vi "Autonomous Independent.vi"   [LabVIEW 2014]
doc: "This VI is called when autonomous begins, and will automatically be terminated when autonomous ends. You can carry out timed or sensor driven robot movement independently without needing to return to the caller."
uses:
  <vilib>/Rock Robotics/WPI/SafetyOutput/WPI_SafetyOutputConfigMenu.ctl
  <vilib>/Rock Robotics/Network Tables/SD Read Number.vi
  Robot Global Data.vi
  <vilib>/Rock Robotics/WPI/RobotDrive/WPI_RobotDriveGetSetRefNum.vi
types:
  T1 = enum16{"Wait 0", "Reta 1", "Wait 1", "Curva 1 ", "Reta 2", "Curva 2", "Reta 3"}
  T2 = enum16{"Get Bin", "Get Tote", "Wait 1", "Release"}
  T3 = typedef "WPI_SafetyOutputConfigMenu.ctl" = enum16{"Enable", "Disable"}
  T4 = enum16{"FALCOOOOOOOON PUNCH 1", "Wait 1", "FALCOOOOOOOON PUNCH 2", "Wait 2"}
  T5 = enum16{"Wait 0", "Reta 1", "Wait 1", "Reta 2", "Wait 2", "Curva 1", "Wait 3", "Reta 3", "Curva 2", "Wait 4", "Reta 4"}
  T6 = enum16{"Get 1st Tote", "Wait 1", "Get 2nd Tote", "Wait 2", "Get 3rd Tote", "Wait 3", "Release"}
  T7 = enum16{"Wait", "Empty state", "Get Bin", "Get Tote First", "Get Knocked Bin", "Close Gripper - Bin", "Close Gripper", "Carry Bin Mode", "Carry Tote Mode", "Get Tote", "Change Height", "Open Gripper", "Get to 0", "Release Pile"}
  T8 = typedef "WPI_EncoderDevRef.ctl" = cluster{"DevStatus":errorcluster, "EncoderIndex":T9, "CounterIndex":T10, "DistancePerCount":dbl, "Decoding Type":T11}
  T9 = typedef "FPGA_EncoderIdx.ctl" = enum8{"Enc 0", "Enc 1", "Enc 2", "Enc 3", "Enc 4", "Enc 5", "Enc 6", "Enc 7", "Invalid"}
  T10 = typedef "FPGA_CounterCtrSystemIndex.ctl" = enum8{"Ctr 0", "Ctr 1", "Ctr 2", "Ctr 3", "Ctr 4", "Ctr 5", "Ctr 6", "Ctr 7", "Invalid"}
  T11 = typedef "WPI_EncoderType.ctl" = enum16{"1x", "2x", "4x"}
  T12 = typedef "WPI_RobotDriveDevRef.ctl" = cluster{"DevStatus":errorcluster, "Motors[]":T13[], "Square Inputs":bool, "Max Output":dbl}
  T13 = typedef "WPI_MotorControlDeviceRef.ctl" = cluster{"DeviceStatus":errorcluster, "Type":T14, "PWM":cluster{"Controller":T15, "PWM Channel":T16, "DeadBand":T17}, "CAN":cluster{"Device Number":u8, "Control Mode":T18, "Semaphore":T19, "Max Vout":dbl, "TalonSRX Control Mode":T20}, "Invert":bool, "TransformRef":T21, "InvTransformRef":T21}
  T14 = typedef "WPI_MotorControlType.ctl" = enum16{"PWM", "CAN", "CANTalonSRX"}
  T15 = typedef "FPGA_TypedefDigitalModule.ctl" = enum16{"Controller 1"}
  T16 = typedef "FPGA_DIOPWMChannel.ctl" = enum8{"PWM 0", "PWM 1", "PWM 2", "PWM 3", "PWM 4", "PWM 5", "PWM 6", "PWM 7", "PWM 8", "PWM 9", "PWM MXP 0", "PWM MXP 1", "PWM MXP 2", "PWM MXP 3", "PWM MXP 4", "PWM MXP 5", "PWM MXP 6", "PWM MXP 7", "PWM MXP 8", "PWM MXP 9", "Invalid"}
  T17 = typedef "WPI_PWMDeadband.ctl" = cluster{"Name":string, "maxPositivePwm":i32, "minPositivePwm":i32, "centerPwm":i32, "maxNegativePwm":i32, "minNegativePwm":i32, "angularRange":u16}
  T18 = typedef "WPI_CANJaguar_ControlMode.ctl" = enum8{"Percent VBus", "Current", "Speed", "Position", "Voltage"}
  T19 = typedef "Semaphore RefNum" = refnum<k1>
  T20 = typedef "WPI_CANTalonSRX_APIControlMode.ctl" = enum8{"Percent VBus", "Speed", "Position", "Slave", "Unchanged / Invalid"}
  T21 = typedef "WPI_PWMTransform_ConPane.ctl" = refnum<vi>
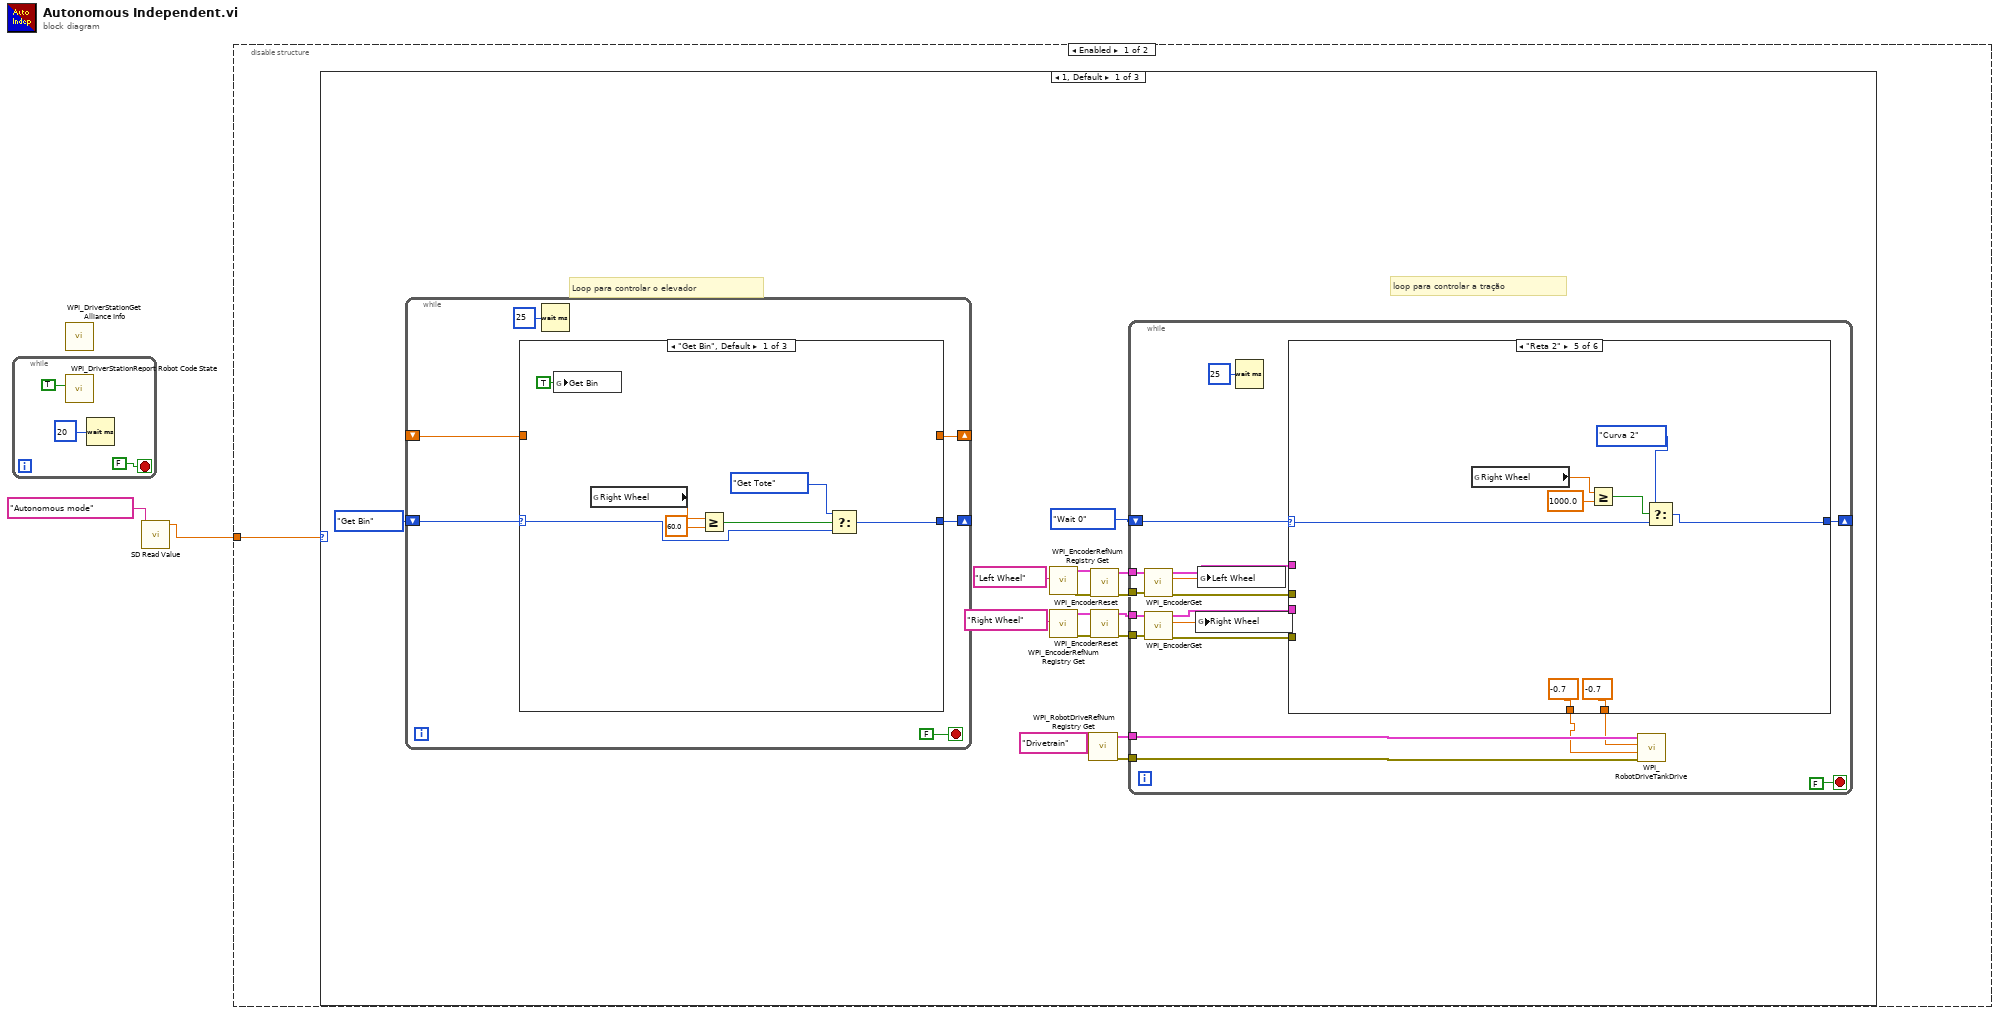
[diagram p0: block diagram]
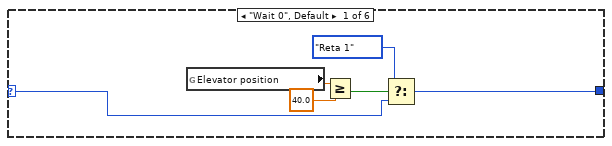
[diagram p2: hidden frame]
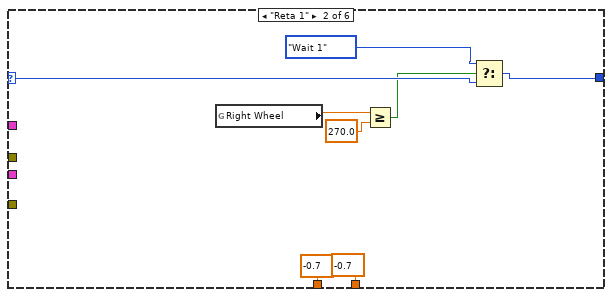
[diagram p3: hidden frame]
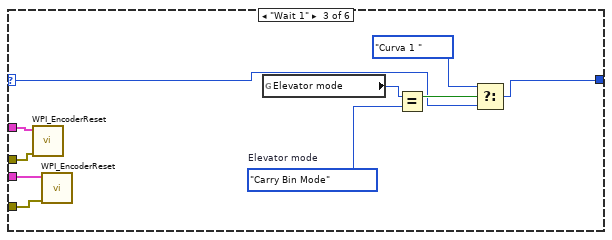
[diagram p4: hidden frame]
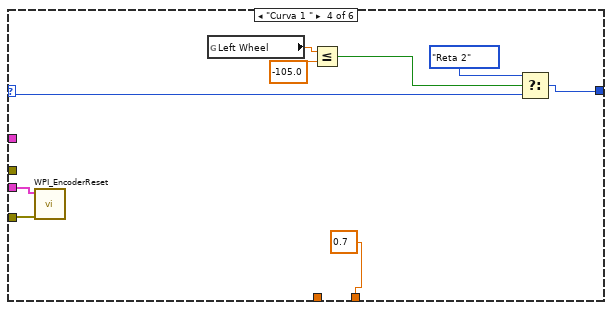
[diagram p5: hidden frame]
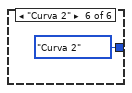
[diagram p6: hidden frame]
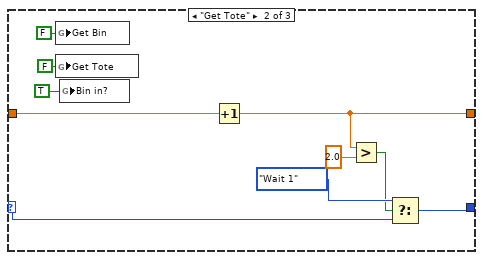
[diagram p7: hidden frame]
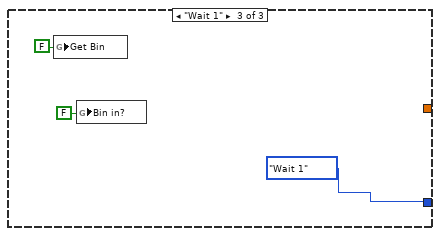
[diagram p8: hidden frame]
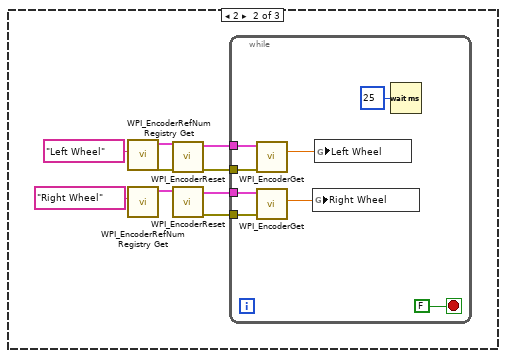
[diagram p9: hidden frame]
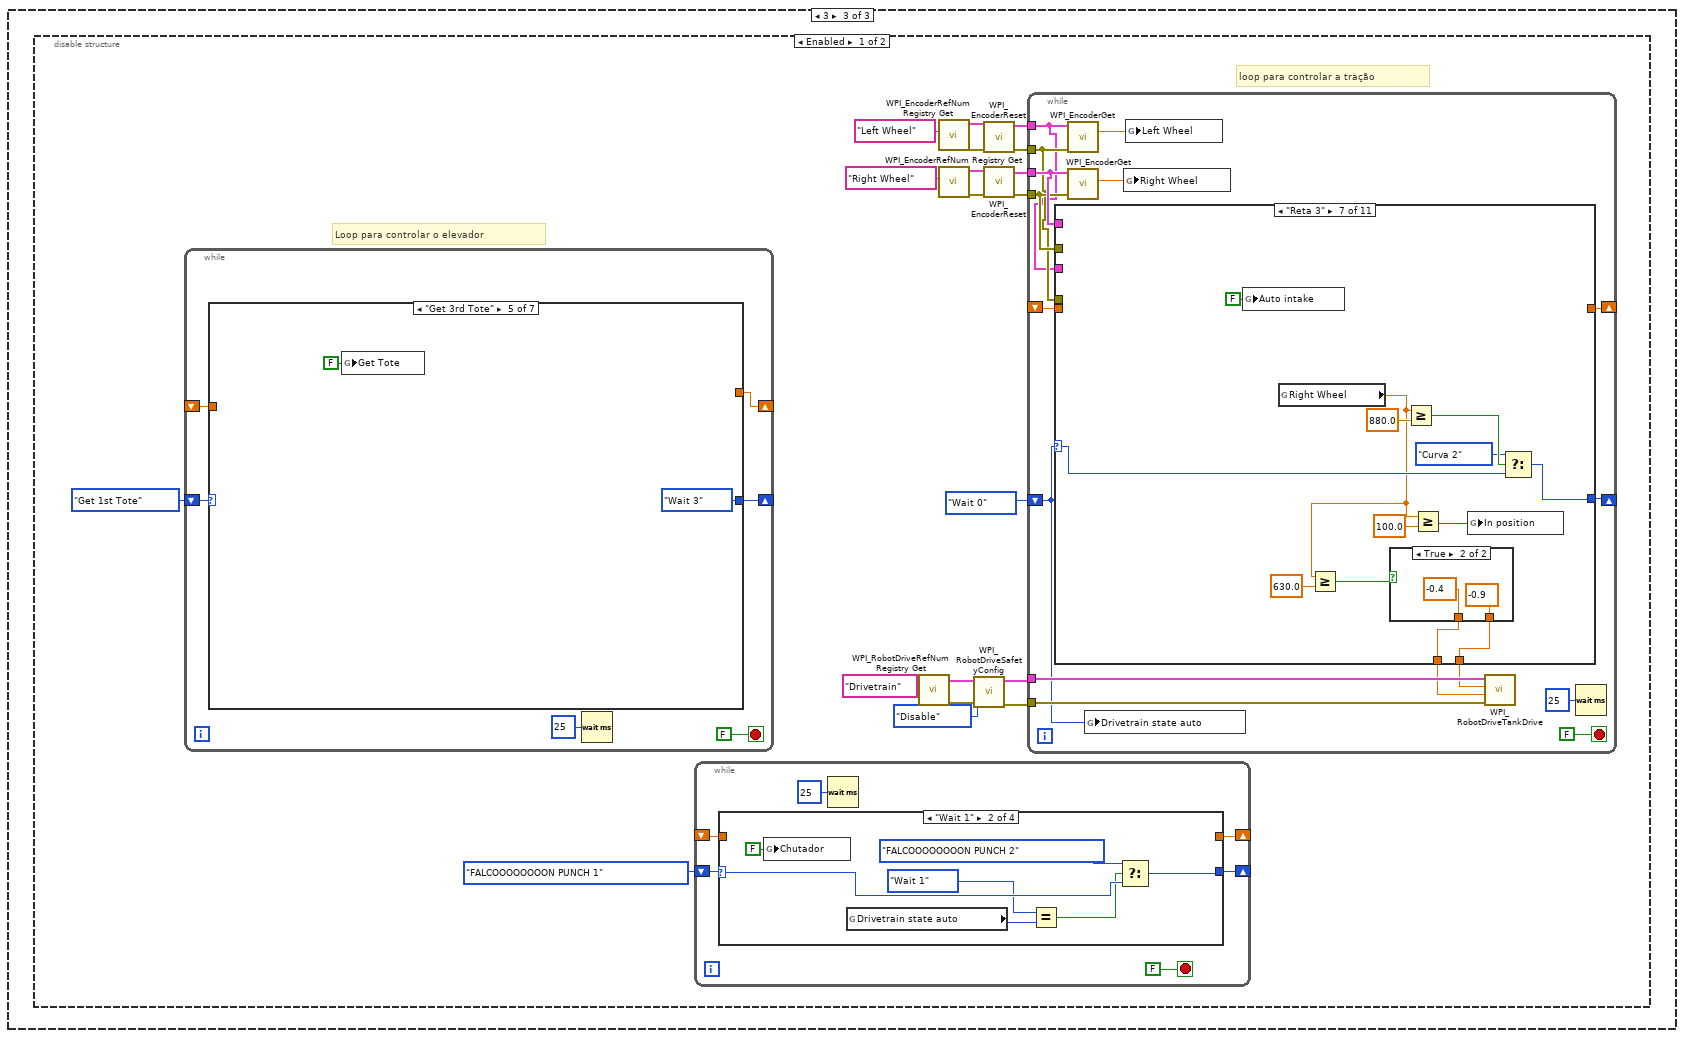
[diagram p10: hidden frame]
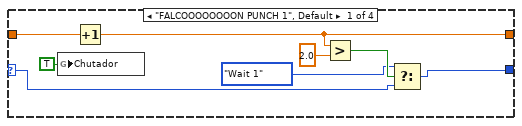
[diagram p11: hidden frame]
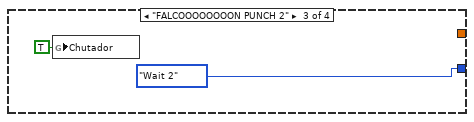
[diagram p12: hidden frame]
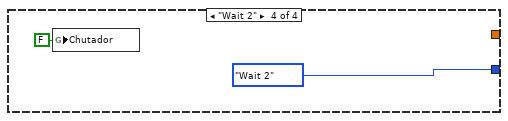
[diagram p13: hidden frame]
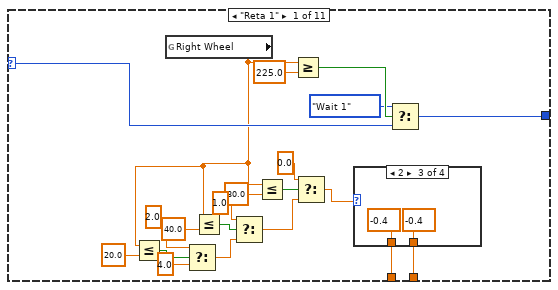
[diagram p14: hidden frame]
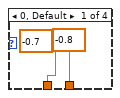
[diagram p15: hidden frame]
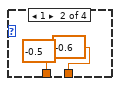
[diagram p16: hidden frame]
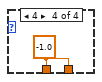
[diagram p17: hidden frame]
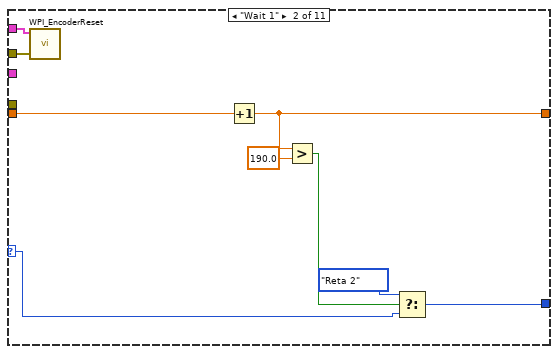
[diagram p18: hidden frame]
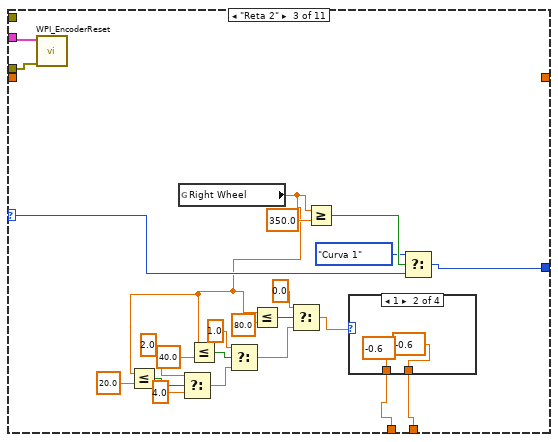
[diagram p19: hidden frame]
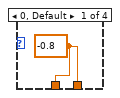
[diagram p20: hidden frame]
diagram:
  n1 = while {
    stop <- FALSE stop-if-true
    n2 = call <vilib>:"WPI_DriverStationReport Robot Code State.vi"("Autonomous"=TRUE) -> ()  [unwired: 10 in, 1 out]
    n3 = Wait (ms)(milliseconds to wait=u32 20) -> ()  [unwired: 1 out]
  }
  n4 = call <vilib>:"WPI_DriverStationGet Alliance Info.vi"() -> ()  [unwired: 12 out]
  n5 = call-poly <vilib>:"SD Read Value.vi"("Name"="Autonomous mode") -> ("Numeric"=w2:dbl)  [unwired: 8 in, 2 out]
  n6 = disable-structure shown="Enabled" {
    disable-tunnel: w2 -> [w6 _]
    frame Enabled {
      n7 = case shown="1, Default" w6 {
        frame 1, Default {
          # "loop para controlar a tração"
          # "Loop para controlar o elevador"
          n8 = while {
            shift-right: [w85] -> _
            shift-left: T2."Get Bin" -> [w82]
            shift-right: [w83] -> _
            shift-left: _ -> [w84]
            stop <- FALSE stop-if-true
            n9 = case shown="\"Get Bin\", Default" w82 {
              selector: w82 -> [w88 w100 _]
              tunnel: [w91 w101 T2."Wait 1"] -> w85
              tunnel: w84 -> [_ w102 _]
              tunnel: [_ w98 _] -> w83
              frame "Get Bin", Default {
                n10 = global write "Robot Global Data.vi" "Get Bin"(TRUE ("Get Bin")) -> ()
                n11 = global read "Robot Global Data.vi" "Right Wheel"() -> (w93:dbl)
                n12 = Greater Or Equal?(x=w93, y=60.0) -> (x >= y?=w89:bool)
                n13 = Select(t=T2."Get Tote", s=w89, f=w88) -> (s? t:f=w91:T2)
              }
              frame "Get Tote" {
                n14 = global write "Robot Global Data.vi" "Get Bin"(FALSE ("Get Bin")) -> ()
                n15 = global write "Robot Global Data.vi" "Get Tote"(FALSE ("Get Tote")) -> ()
                n16 = global write "Robot Global Data.vi" "Bin in?"(TRUE ("Get Tote")) -> ()
                n17 = Increment(x=w102) -> (x+1=w98:dbl)
                n18 = Greater?(x=w98, y=2.0) -> (0:w96:bool)
                n19 = Select(t=T2."Wait 1", s=w96, f=w100) -> (s? t:f=w101:T2)
              }
              frame "Wait 1" {
                n20 = global write "Robot Global Data.vi" "Get Bin"(FALSE ("Get Bin")) -> ()
                n21 = global write "Robot Global Data.vi" "Bin in?"(FALSE ("Bin in?")) -> ()
              }
            }
            n22 = Wait (ms)(milliseconds to wait=u32 25) -> ()  [unwired: 1 out]
          }
          n23 = call <vilib>:"WPI_EncoderRefNum Registry Get.vi"("refnum name"="Left Wheel") -> ("error out"=w7:errorcluster, "EncoderDevRef"=w8:T8)  [unwired: 9 in]
          n24 = call <vilib>:"WPI_EncoderRefNum Registry Get.vi"("refnum name"="Right Wheel") -> ("error out"=w14:errorcluster, "EncoderDevRef"=w13:T8)  [unwired: 9 in]
          n25 = call <vilib>:"WPI_RobotDriveRefNum Registry Get.vi"("refnum name"="Drivetrain") -> ("error out"=w15:errorcluster, "RobotDriveDevRef"=w16:T12)  [unwired: 9 in]
          n26 = call <vilib>:"WPI_EncoderReset.vi"("error in (no error)"=w7, "EncoderDevRef"=w8) -> ("error out"=w10:errorcluster, "EncoderDevRef"=w9:T8)  [unwired: 8 in]
          n27 = call <vilib>:"WPI_EncoderReset.vi"("error in (no error)"=w14, "EncoderDevRef"=w13) -> ("error out"=w11:errorcluster, "EncoderDevRef"=w12:T8)  [unwired: 8 in]
          n28 = while {
            shift-right: [w30] -> _
            shift-left: T1."Wait 0" -> [w38]
            tunnel: w9 -> [w37]
            tunnel: w10 -> [w36]
            tunnel: w12 -> [w35]
            tunnel: w11 -> [w34]
            tunnel: w16 -> [w29]
            tunnel: w15 -> [w28]
            stop <- FALSE stop-if-true
            n29 = call <vilib>:"WPI_EncoderGet.vi"("error in (no error)"=w36, "EncoderDevRef"=w37) -> ("error out"=w25:errorcluster, "Distance"=w33:dbl, "EncoderDevRef"=w24:T8)  [unwired: 4 in, 3 out]
            n30 = call <vilib>:"WPI_EncoderGet.vi"("error in (no error)"=w34, "EncoderDevRef"=w35) -> ("error out"=w26:errorcluster, "Distance"=w32:dbl, "EncoderDevRef"=w27:T8)  [unwired: 4 in, 3 out]
            n31 = global write "Robot Global Data.vi" "Right Wheel"(w32) -> ()
            n32 = global write "Robot Global Data.vi" "Left Wheel"(w33) -> ()
            n33 = Wait (ms)(milliseconds to wait=u32 25) -> ()  [unwired: 1 out]
            n34 = case shown="\"Reta 2\"" w38 {
              selector: w38 -> [w41 w49 w60 w70 w74 _]
              tunnel: [w42 w50 w61 w72 w73 T1."Curva 2" ("t")] -> w30
              tunnel: [_ -0.7 ("Left axis value") _ 0.7 ("Left axis value") -0.7 ("Left axis value") _] -> w23
              tunnel: [_ -0.7 ("Left axis value") _ _ -0.7 ("Left axis value") _] -> w22
              tunnel: w27 -> [_ _ w58 w64 _ _]
              tunnel: w26 -> [_ _ w57 w65 _ _]
              tunnel: w25 -> [_ _ w56 _ _ _]
              tunnel: w24 -> [_ _ w55 _ _ _]
              frame "Wait 0", Default {
                n35 = global read "Robot Global Data.vi" "Elevator position"() -> (w45:dbl)
                n36 = Greater Or Equal?(x=w45, y=40.0) -> (x >= y?=w43:bool)
                n37 = Select(t=T1."Reta 1", s=w43, f=w41) -> (s? t:f=w42:T1)
              }
              frame "Reta 1" {
                n38 = global read "Robot Global Data.vi" "Right Wheel"() -> (w48:dbl)
                n39 = Greater Or Equal?(x=w48, y=270.0) -> (x >= y?=w46:bool)
                n40 = Select(t=T1."Wait 1", s=w46, f=w49) -> (s? t:f=w50:T1)
              }
              frame "Wait 1" {
                w54 = T7."Carry Bin Mode"  # Elevator mode
                n41 = call <vilib>:"WPI_EncoderReset.vi"("error in (no error)"=w56, "EncoderDevRef"=w55) -> ()  [unwired: 8 in, 2 out]
                n42 = call <vilib>:"WPI_EncoderReset.vi"("error in (no error)"=w57, "EncoderDevRef"=w58) -> ()  [unwired: 8 in, 2 out]
                n43 = global read "Robot Global Data.vi" "Elevator mode"() -> (w63:T7)
                n44 = Equal?(x=w63, y=w54) -> (x = y?=w62:bool)
                n45 = Select(t=T1."Curva 1 ", s=w62, f=w60) -> (s? t:f=w61:T1)
              }
              frame "Curva 1 " {
                n46 = call <vilib>:"WPI_EncoderReset.vi"("error in (no error)"=w65, "EncoderDevRef"=w64) -> ()  [unwired: 8 in, 2 out]
                n47 = global read "Robot Global Data.vi" "Left Wheel"() -> (w68:dbl)
                n48 = Less Or Equal?(x=w68, y=-105.0) -> (x <= y?=w66:bool)
                n49 = Select(t=T1."Reta 2", s=w66, f=w70) -> (s? t:f=w72:T1)
              }
              frame "Reta 2" {
                n50 = global read "Robot Global Data.vi" "Right Wheel"() -> (w77:dbl)
                n51 = Greater Or Equal?(x=w77, y=1000.0) -> (x >= y?=w76:bool)
                n52 = Select(t=T1."Curva 2", s=w76, f=w74) -> (s? t:f=w73:T1)
              }
              frame "Curva 2" {
              }
            }
            n53 = call <vilib>:"WPI_RobotDriveTankDrive.vi"("error in (no error)"=w28, "Right axis value"=w22, "Left axis value"=w23, "RobotDriveDevRef"=w29) -> ()  [unwired: 5 in, 3 out]
          }
        }
        frame 2 {
          n54 = call <vilib>:"WPI_EncoderRefNum Registry Get.vi"("refnum name"="Left Wheel") -> ("error out"=w116:errorcluster, "EncoderDevRef"=w115:T8)  [unwired: 9 in]
          n55 = call <vilib>:"WPI_EncoderRefNum Registry Get.vi"("refnum name"="Right Wheel") -> ("EncoderDevRef"=w114:T8)  [unwired: 9 in, 1 out]
          n56 = call <vilib>:"WPI_EncoderReset.vi"("error in (no error)"=w116, "EncoderDevRef"=w115) -> ("error out"=w110:errorcluster, "EncoderDevRef"=w111:T8)  [unwired: 8 in]
          n57 = call <vilib>:"WPI_EncoderReset.vi"("EncoderDevRef"=w114) -> ("error out"=w108:errorcluster, "EncoderDevRef"=w109:T8)  [unwired: 9 in]
          n58 = while {
            tunnel: w111 -> [w121]
            tunnel: w110 -> [w120]
            tunnel: w109 -> [w119]
            tunnel: w108 -> [w118]
            stop <- FALSE stop-if-true
            n59 = call <vilib>:"WPI_EncoderGet.vi"("error in (no error)"=w120, "EncoderDevRef"=w121) -> ("Distance"=w124:dbl)  [unwired: 4 in, 5 out]
            n60 = call <vilib>:"WPI_EncoderGet.vi"("error in (no error)"=w118, "EncoderDevRef"=w119) -> ("Distance"=w123:dbl)  [unwired: 4 in, 5 out]
            n61 = global write "Robot Global Data.vi" "Right Wheel"(w123) -> ()
            n62 = global write "Robot Global Data.vi" "Left Wheel"(w124) -> ()
            n63 = Wait (ms)(milliseconds to wait=u32 25) -> ()  [unwired: 1 out]
          }
        }
        frame 3 {
          n64 = disable-structure shown="Enabled" {
            frame Enabled {
              # "loop para controlar a tração"
              # "Loop para controlar o elevador"
              n65 = while {
                shift-right: [w309] -> _
                shift-left: T6."Get 1st Tote" -> [w311]
                shift-right: [w308] -> _
                shift-left: _ -> [w307]
                stop <- FALSE stop-if-true
                n66 = case shown="\"Get 3rd Tote\"" w311 {
                  selector: w311 -> [w313 w326 w331 w339 _ w349 _]
                  tunnel: [w314 w328 w333 w340 T6."Wait 3" w350 T6."Release"] -> w309
                  tunnel: [w317 _ w334 _ _ _ _] -> w308
                  tunnel: w307 -> [w318 _ w335 _ _ _ _]
                  frame "Get 1st Tote", Default {
                    n67 = global write "Robot Global Data.vi" "Get Tote"(TRUE ("Get Tote")) -> ()
                    n68 = Increment(x=w318) -> (x+1=w317:dbl)
                    n69 = Greater Or Equal?(x=w317, y=30.0) -> (x >= y?=w316:bool)
                    n70 = Select(t=T6."Wait 1", s=w316, f=w313) -> (s? t:f=w314:T6)
                  }
                  frame "Wait 1" {
                    n71 = global write "Robot Global Data.vi" "Get Tote"(TRUE ("Get Tote")) -> ()
                    n72 = global read "Robot Global Data.vi" "Elevator mode"() -> (w325:T7)
                    n73 = global write "Robot Global Data.vi" "Auto intake"(FALSE ("Auto intake")) -> ()
                    n74 = global write "Robot Global Data.vi" "Solenoide"(FALSE ("Auto intake")) -> ()
                    n75 = Equal?(x=w325, y=T7."Carry Tote Mode") -> (x = y?=w323:bool)
                    n76 = Select(t=T6."Get 2nd Tote", s=w323, f=w326) -> (s? t:f=w328:T6)
                  }
                  frame "Get 2nd Tote" {
                    n77 = Increment(x=w335) -> (x+1=w334:dbl)
                    n78 = global write "Robot Global Data.vi" "Get Tote"(TRUE ("Get Tote")) -> ()
                    n79 = Greater Or Equal?(x=w334, y=15.0) -> (x >= y?=w330:bool)
                    n80 = Select(t=T6."Wait 2", s=w330, f=w331) -> (s? t:f=w333:T6)
                  }
                  frame "Wait 2" {
                    n81 = global write "Robot Global Data.vi" "Get Tote"(FALSE ("Get Tote")) -> ()
                    n82 = global read "Robot Global Data.vi" "Elevator mode"() -> (w342:T7)
                    n83 = Equal?(x=w342, y=T7."Carry Tote Mode") -> (x = y?=w338:bool)
                    n84 = Select(t=T6."Get 3rd Tote", s=w338, f=w339) -> (s? t:f=w340:T6)
                  }
                  frame "Get 3rd Tote" {
                    n85 = global write "Robot Global Data.vi" "Get Tote"(FALSE ("Get Tote")) -> ()
                  }
                  frame "Wait 3" {
                    n86 = global write "Robot Global Data.vi" "Get Tote"(FALSE ("Get Tote")) -> ()
                    n87 = global read "Robot Global Data.vi" "In position"() -> (w348:bool)
                    n88 = Select(t=T6."Release", s=w348, f=w349) -> (s? t:f=w350:T6)
                  }
                  frame "Release" {
                    n89 = global write "Robot Global Data.vi" "Release"(TRUE ("Release")) -> ()
                  }
                }
                n90 = Wait (ms)(milliseconds to wait=u32 25) -> ()  [unwired: 1 out]
              }
              n91 = while {
                shift-right: [w146] -> _
                shift-left: T4."FALCOOOOOOOON PUNCH 1" -> [w148]
                shift-right: [w144] -> _
                shift-left: _ -> [w145]
                stop <- FALSE stop-if-true
                n92 = case shown="\"Wait 1\"" w148 {
                  selector: w148 -> [w151 w162 _ _]
                  tunnel: [w153 w163 T4."Wait 2" T4."Wait 2"] -> w146
                  tunnel: w145 -> [w156 _ _ _]
                  tunnel: [w155 _ _ _] -> w144
                  frame "FALCOOOOOOOON PUNCH 1", Default {
                    n93 = global write "Robot Global Data.vi" "Chutador"(TRUE ("Chutador")) -> ()
                    n94 = Increment(x=w156) -> (x+1=w155:dbl)
                    n95 = Greater?(x=w155, y=2.0) -> (0:w152:bool)
                    n96 = Select(t=T4."Wait 1", s=w152, f=w151) -> (s? t:f=w153:T4)
                  }
                  frame "Wait 1" {
                    n97 = global write "Robot Global Data.vi" "Chutador"(FALSE ("Chutador")) -> ()
                    n98 = global read "Robot Global Data.vi" "Drivetrain state auto"() -> (w160:T5)
                    n99 = Equal?(x=T5."Wait 1", y=w160) -> (x = y?=w158:bool)
                    n100 = Select(t=T4."FALCOOOOOOOON PUNCH 2", s=w158, f=w162) -> (s? t:f=w163:T4)
                  }
                  frame "FALCOOOOOOOON PUNCH 2" {
                    n101 = global write "Robot Global Data.vi" "Chutador"(TRUE ("Chutador")) -> ()
                  }
                  frame "Wait 2" {
                    n102 = global write "Robot Global Data.vi" "Chutador"(FALSE ("Chutador")) -> ()
                  }
                }
                n103 = Wait (ms)(milliseconds to wait=u32 25) -> ()  [unwired: 1 out]
              }
              n104 = call <vilib>:"WPI_RobotDriveRefNum Registry Get.vi"("refnum name"="Drivetrain") -> ("error out"=w128:errorcluster, "RobotDriveDevRef"=w129:T12)  [unwired: 9 in]
              n105 = call <vilib>:"WPI_EncoderRefNum Registry Get.vi"("refnum name"="Left Wheel") -> ("error out"=w139:errorcluster, "EncoderDevRef"=w138:T8)  [unwired: 9 in]
              n106 = call <vilib>:"WPI_EncoderRefNum Registry Get.vi"("refnum name"="Right Wheel") -> ("error out"=w136:errorcluster, "EncoderDevRef"=w137:T8)  [unwired: 9 in]
              n107 = call <vilib>:"WPI_RobotDriveSafetyConfig.vi"("error in (no error)"=w128, "mode"=WPI_SafetyOutputConfigMenu."Disable", "RobotDriveDevRef"=w129) -> ("error out"=w126:errorcluster, "RobotDriveDevRef"=w127:T12)  [unwired: 7 in]
              n108 = call <vilib>:"WPI_EncoderReset.vi"("error in (no error)"=w139, "EncoderDevRef"=w138) -> ("error out"=w132:errorcluster, "EncoderDevRef"=w133:T8)  [unwired: 8 in]
              n109 = call <vilib>:"WPI_EncoderReset.vi"("error in (no error)"=w136, "EncoderDevRef"=w137) -> ("error out"=w130:errorcluster, "EncoderDevRef"=w131:T8)  [unwired: 8 in]
              n110 = while {
                shift-right: [w180] -> _
                shift-left: T5."Wait 0" -> [w175]
                tunnel: w127 -> [w182]
                tunnel: w126 -> [w181]
                tunnel: w133 -> [w169]
                tunnel: w132 -> [w170]
                tunnel: w131 -> [w172]
                tunnel: w130 -> [w171]
                shift-right: [w176] -> _
                shift-left: _ -> [w177]
                stop <- FALSE stop-if-true
                n111 = case shown="\"Reta 3\"" w175 {
                  selector: w175 -> [w204 w219 w240 _ w259 _ w278 _ w294 _ w305]
                  tunnel: [w199 _ w225 _ 0.7 ("y") _ w270 _ w292 _ _] -> w174
                  tunnel: [w205 w218 w241 T5."Curva 1" w261 T5."Reta 3" w279 T5."Wait 4" w293 T5."Reta 4" w306] -> w180
                  tunnel: w177 -> [_ w217 _ _ _ _ _ _ _ _ w303]
                  tunnel: [_ w216 _ _ _ _ _ _ _ _ w302] -> w176
                  tunnel: [w198 _ w226 _ -0.7 ("y") _ w271 _ w292 _ _] -> w173
                  tunnel: w172 -> [_ w213 _ _ _ w268 _ w290 _ _ _]
                  tunnel: w171 -> [_ w214 _ _ _ w267 _ w289 _ _ _]
                  tunnel: w170 -> [_ _ w222 w253 _ w266 _ w287 _ _ _]
                  tunnel: w169 -> [_ _ w223 w252 _ w265 _ w288 _ _ _]
                  frame "Reta 1" {
                    n112 = global read "Robot Global Data.vi" "Right Wheel"() -> (w187:dbl)
                    n113 = Less Or Equal?(x=w187, y=20.0) -> (x <= y?=w189:bool)
                    n114 = Select(t=2.0, s=w189, f=4.0) -> (s? t:f=w190:dbl)
                    n115 = Less Or Equal?(x=w187, y=40.0) -> (x <= y?=w193:bool)
                    n116 = Select(t=1.0, s=w193, f=w190) -> (s? t:f=w192:dbl)
                    n117 = Less Or Equal?(x=w187, y=80.0) -> (x <= y?=w197:bool)
                    n118 = Greater Or Equal?(x=w187, y=225.0) -> (x >= y?=w203:bool)
                    n119 = Select(t=0.0, s=w197, f=w192) -> (s? t:f=w195:dbl)
                    n120 = case shown="2" w195 {
                      tunnel: [-0.7 ("y") -0.5 ("y") -0.4 ("y") w212] -> w199
                      tunnel: [-0.8 ("y") -0.6 ("y") -0.4 ("y") w212] -> w198
                      frame 0, Default {
                      }
                      frame 1 {
                      }
                      frame 2 {
                      }
                      frame 4 {
                        w212 = -1.0 ("y")
                      }
                    }
                    n121 = Select(t=T5."Wait 1", s=w203, f=w204) -> (s? t:f=w205:T5)
                  }
                  frame "Wait 1" {
                    n122 = call <vilib>:"WPI_EncoderReset.vi"("error in (no error)"=w214, "EncoderDevRef"=w213) -> ()  [unwired: 8 in, 2 out]
                    n123 = Increment(x=w217) -> (x+1=w216:dbl)
                    n124 = Greater?(x=w216, y=190.0) -> (0:w215:bool)
                    n125 = Select(t=T5."Reta 2", s=w215, f=w219) -> (s? t:f=w218:T5)
                  }
                  frame "Reta 2" {
                    n126 = call <vilib>:"WPI_EncoderReset.vi"("error in (no error)"=w222, "EncoderDevRef"=w223) -> ()  [unwired: 8 in, 2 out]
                    n127 = global read "Robot Global Data.vi" "Right Wheel"() -> (w224:dbl)
                    n128 = Less Or Equal?(x=w224, y=20.0) -> (x <= y?=w230:bool)
                    n129 = Select(t=2.0, s=w230, f=4.0) -> (s? t:f=w231:dbl)
                    n130 = Less Or Equal?(x=w224, y=40.0) -> (x <= y?=w234:bool)
                    n131 = Select(t=1.0, s=w234, f=w231) -> (s? t:f=w233:dbl)
                    n132 = Less Or Equal?(x=w224, y=80.0) -> (x <= y?=w238:bool)
                    n133 = Select(t=0.0, s=w238, f=w233) -> (s? t:f=w236:dbl)
                    n134 = Greater Or Equal?(x=w224, y=350.0) -> (x >= y?=w244:bool)
                    n135 = case shown="1" w236 {
                      tunnel: [w245 -0.6 ("y") -0.35 ("y") w250] -> w225
                      tunnel: [w245 -0.6 ("y") -0.4 ("y") w250] -> w226
                      frame 0, Default {
                        w245 = -0.8 ("y")
                      }
                      frame 1 {
                      }
                      frame 2 {
                      }
                      frame 4 {
                        w250 = -1.0 ("y")
                      }
                    }
                    n136 = Select(t=T5."Curva 1", s=w244, f=w240) -> (s? t:f=w241:T5)
                  }
                  frame "Wait 2" {
                    n137 = call <vilib>:"WPI_EncoderReset.vi"("error in (no error)"=w253, "EncoderDevRef"=w252) -> ()  [unwired: 8 in, 2 out]
                    n138 = global write "Robot Global Data.vi" "Auto intake"(FALSE ("Auto intake")) -> ()
                  }
                  frame "Curva 1" {
                    n139 = global read "Robot Global Data.vi" "Left Wheel"() -> (w258:dbl)
                    n140 = global write "Robot Global Data.vi" "Auto intake"(TRUE ("Auto intake")) -> ()
                    n141 = Greater Or Equal?(x=w258, y=90.0) -> (x >= y?=w256:bool)
                    n142 = Select(t=T5."Wait 3", s=w256, f=w259) -> (s? t:f=w261:T5)
                  }
                  frame "Wait 3" {
                    n143 = call <vilib>:"WPI_EncoderReset.vi"("error in (no error)"=w266, "EncoderDevRef"=w265) -> ()  [unwired: 8 in, 2 out]
                    n144 = call <vilib>:"WPI_EncoderReset.vi"("error in (no error)"=w267, "EncoderDevRef"=w268) -> ()  [unwired: 8 in, 2 out]
                    n145 = global write "Robot Global Data.vi" "Auto intake"(FALSE ("Auto intake")) -> ()
                  }
                  frame "Reta 3" {
                    n146 = global write "Robot Global Data.vi" "Auto intake"(FALSE ("Auto intake")) -> ()
                    n147 = global read "Robot Global Data.vi" "Right Wheel"() -> (w272:dbl)
                    n148 = Greater Or Equal?(x=w272, y=630.0) -> (x >= y?=w273:bool)
                    n149 = case shown="True" w273 {
                      tunnel: [-1.0 ("y") -0.9 ("y")] -> w271
                      tunnel: [-1.0 ("y") -0.4 ("y")] -> w270
                      frame False {
                      }
                      frame True {
                      }
                    }
                    n150 = Greater Or Equal?(x=w272, y=880.0) -> (x >= y?=w282:bool)
                    n151 = Greater Or Equal?(x=w272, y=100.0) -> (x >= y?=w276:bool)
                    n152 = global write "Robot Global Data.vi" "In position"(w276) -> ()
                    n153 = Select(t=T5."Curva 2", s=w282, f=w278) -> (s? t:f=w279:T5)
                  }
                  frame "Curva 2" {
                    n154 = call <vilib>:"WPI_EncoderReset.vi"("error in (no error)"=w289, "EncoderDevRef"=w290) -> ()  [unwired: 8 in, 2 out]
                    n155 = call <vilib>:"WPI_EncoderReset.vi"("error in (no error)"=w287, "EncoderDevRef"=w288) -> ()  [unwired: 8 in, 2 out]
                  }
                  frame "Wait 4" {
                    w292 = 1.0 ("y")
                    n156 = global read "Robot Global Data.vi" "Right Wheel"() -> (w295:dbl)
                    n157 = Less Or Equal?(x=w295, y=-30.0) -> (x <= y?=w298:bool)
                    n158 = Select(t=T5."Reta 4", s=w298, f=w294) -> (s? t:f=w293:T5)
                  }
                  frame "Reta 4" {
                  }
                  frame "Wait 0", Default {
                    n159 = Increment(x=w303) -> (x+1=w302:dbl)
                    n160 = Greater?(x=w302, y=140.0) -> (0:w300:bool)
                    n161 = Select(t=T5."Reta 1", s=w300, f=w305) -> (s? t:f=w306:T5)
                  }
                }
                n162 = call <vilib>:"WPI_EncoderGet.vi"("error in (no error)"=w170, "EncoderDevRef"=w169) -> ("Distance"=w179:dbl)  [unwired: 4 in, 5 out]
                n163 = call <vilib>:"WPI_EncoderGet.vi"("error in (no error)"=w171, "EncoderDevRef"=w172) -> ("Distance"=w178:dbl)  [unwired: 4 in, 5 out]
                n164 = global write "Robot Global Data.vi" "Drivetrain state auto"(w175) -> ()
                n165 = global write "Robot Global Data.vi" "Right Wheel"(w178) -> ()
                n166 = global write "Robot Global Data.vi" "Left Wheel"(w179) -> ()
                n167 = call <vilib>:"WPI_RobotDriveTankDrive.vi"("error in (no error)"=w181, "Right axis value"=w174, "Left axis value"=w173, "RobotDriveDevRef"=w182) -> ()  [unwired: 5 in, 3 out]
                n168 = Wait (ms)(milliseconds to wait=u32 25) -> ()  [unwired: 1 out]
              }
            }
            frame Disabled {
            }
          }
        }
      }
    }
    frame Disabled {
    }
  }
